vi "_init.vi"(8 "error in (no error)":errorcluster, 10 "a_Port":i16, 11 "UV-VIS_AVANTES in":refnum<class "UV-VIS_AVANTES.lvclass">) -> (0 "error out":errorcluster, 2 "number of spectrometers":i32, 3 "UV-VIS_AVANTES out":refnum<class "UV-VIS_AVANTES.lvclass">)   [LabVIEW 2020, in "UV-VIS_AVANTES.lvclass"]
uses:
  UV-VIS_AVANTES.lvclass
  C:/dev/TRANCON/Classes/Detector/Detector.lvclass
  Detector.lvclass/Detector.ctl
  Detector.lvclass
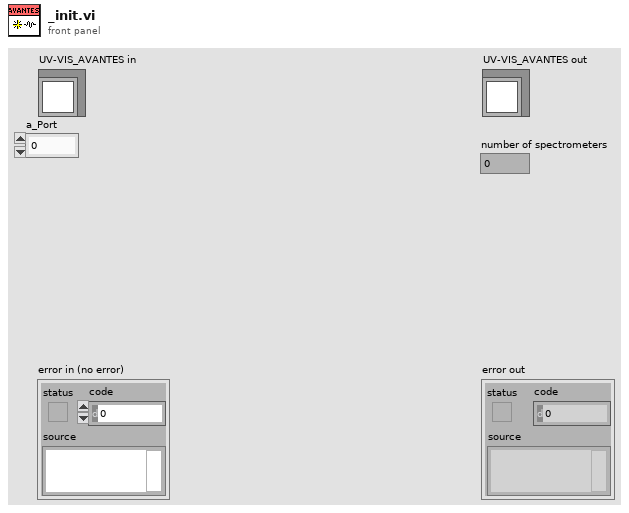
[diagram p1: front panel]
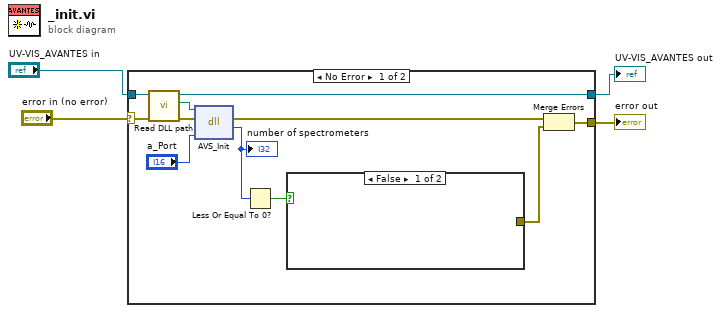
[diagram p0: block diagram]
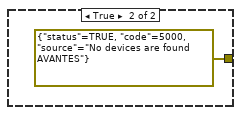
[diagram p2: hidden frame]
diagram:
  n1 = case shown="No Error" "error in (no error)" {
    selector: "error in (no error)" -> [w14 w18]
    tunnel: [w5 w18] -> w3
    tunnel: [w13 w17] -> w1
    tunnel: "UV-VIS_AVANTES in" -> [w15 w17]
    frame No Error {
      n2 = call "Read DLL path.vi"("error in (no error)"=w14, "Detector in"=w15) -> ("error out"=w12:errorcluster, "DLL path"=w11:path, "Detector out"=w13:refnum<class "UV-VIS_AVANTES.lvclass">)  [unwired: 7 in]
      n3 = dll-call lib="C:/AvaSpecX64-DLL_9.4/examples/LabView/LabViewSingleChan/avaspec.dll" fn="AVS_Init"(path in=w11, error in=w12, "a_Port"="a_Port") -> (error out=w6:errorcluster, "return type"=w9:i32)  [unwired: 2 in, 1 out]
      "number of spectrometers" <- w9
      n4 = Less Or Equal To 0?(x=w9) -> (x <= 0?=w8:bool)
      n5 = case shown="False" w8 {
        tunnel: [_ errorcluster {"status"=TRUE, "code"=5000, "source"="No devices are found AVANTES"} ("error in (no error)")] -> w7
        frame False {
        }
        frame True {
        }
      }
      n6 = Merge Errors(w6, w7) -> (w5:errorcluster)
    }
    frame Error {
    }
  }
  "error out" <- w3
  "UV-VIS_AVANTES out" <- w1
